vi "6.3 Cluster retrieve with 2D Array elements.vi"() -> ()   [LabVIEW 2017]
uses:
  1b87943d-a1ca-48d8-8490-e1b7ad6daeb6.vi
  da318448-3cad-42ed-b567-b1a7b9d2dcdc.vi
  API-String-Arugments-Support/_Support/Convert API String Arguments to Data(variant).vi
panel:
  out "output cluster 2":T1={"String"="BoolArray:[0,1,0,1;1,0,1,0;0,1,0,1];Cluster.Boolean:on", "Reference Cluster"={"String"="abc", "BoolArray"=[[FALSE, TRUE, FALSE, TRUE], [TRUE, FALSE, TRUE, FALSE], [FALSE, TRUE, FALSE, TRUE]], "Cluster"={"Boolean"=FALSE}}, "Retrieved Cluster"={"String"="abc", "BoolArray"=[[FALSE, TRUE, FALSE, TRUE], [TRUE, FALSE, TRUE, FALSE], [FALSE, TRUE, FALSE, TRUE]], "Cluster"={"Boolean"=TRUE}}}
  out "output cluster":T1={"String"="BoolArray:[TRUE,FALSE,TRUE,FALSE;FALSE,TRUE,FALSE,TRUE;TRUE,FALSE,TRUE,FALSE]", "Reference Cluster"={"String"="abc", "BoolArray"=[[FALSE, TRUE, FALSE, TRUE], [TRUE, FALSE, TRUE, FALSE], [FALSE, TRUE, FALSE, TRUE]], "Cluster"={"Boolean"=FALSE}}, "Retrieved Cluster"={"String"="abc", "BoolArray"=[[TRUE, FALSE, TRUE, FALSE], [FALSE, TRUE, FALSE, TRUE], [TRUE, FALSE, TRUE, FALSE]], "Cluster"={"Boolean"=FALSE}}}
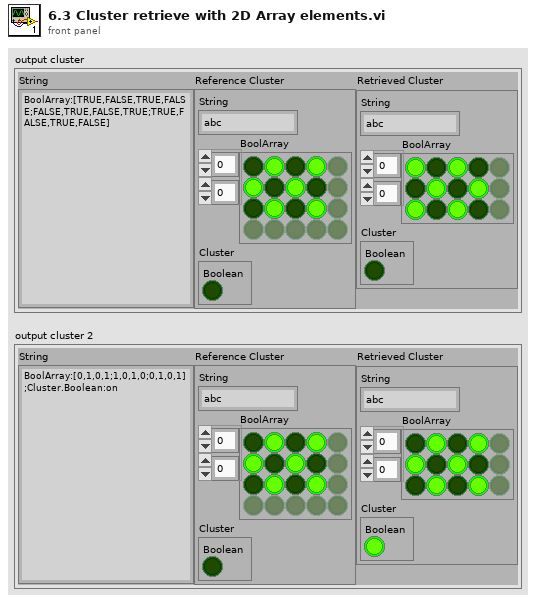
[diagram p1: front panel]
types:
  T1 = cluster{"String":string, "Reference Cluster":cluster{"String":string, "BoolArray":bool[][], "Cluster":cluster{"Boolean":bool}}, "Retrieved Cluster":cluster{"String":string, "BoolArray":bool[][], "Cluster":cluster{"Boolean":bool}}}
  T2 = cluster{"String":string, "BoolArray":bool[][], "Cluster":cluster{"Boolean":bool}}
  T3 = cluster{"String":string, "Cluster":cluster{"String":string, "BoolArray":bool[][], "Cluster":cluster{"Boolean":bool}}, "Data":cluster{"String":string, "BoolArray":bool[][], "Cluster":cluster{"Boolean":bool}}}
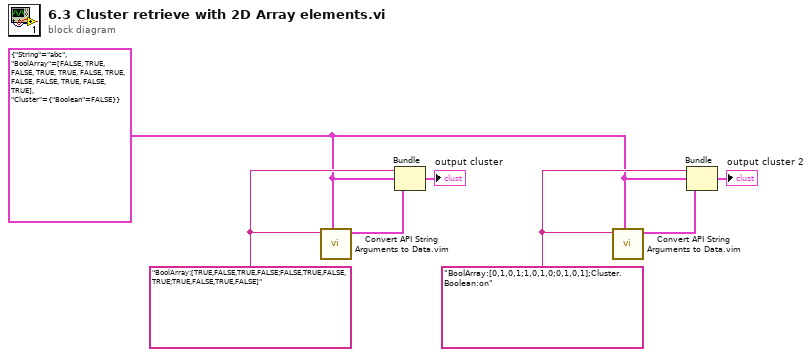
[diagram p0: block diagram]
diagram:
  w4 = "BoolArray:[0,1,0,1;1,0,1,0;0,1,0,1];Cluster.Boolean:on" ("String")
  w5 = "BoolArray:[TRUE,FALSE,TRUE,FALSE;FALSE,TRUE,FALSE,TRUE;TRUE,FALSE,TRUE,FALSE]" ("String")
  w1 = T2 {"String"="abc", "BoolArray"=[[FALSE, TRUE, FALSE, TRUE], [TRUE, FALSE, TRUE, FALSE], [FALSE, TRUE, FALSE, TRUE]], "Cluster"={"Boolean"=FALSE}} ("Cluster")
  n1 = call "Convert API String Arguments to Data.vim"("Type"=w1, "String"=w5) -> ("Data"=w6:T2)  [unwired: 6 in, 1 out]
  n2 = Bundle("String"=w5, "Cluster"=w1, "Data"=w6) -> (→"output cluster":T3)  [unwired: 1 in]
  n3 = call "Convert API String Arguments to Data.vim"("Type"=w1, "String"=w4) -> ("Data"=w3:T2)  [unwired: 6 in, 1 out]
  n4 = Bundle("String"=w4, "Cluster"=w1, "Data"=w3) -> (→"output cluster 2":T3)  [unwired: 1 in]
